vi "Get Delay After FPGA Load.vi"(8 "error in":errorcluster, 11 "scan engine custom device ref in":T1 format="%.0x") -> (0 "error out":errorcluster, 2 "delay after FPGA load (s)":u16, 3 "scan engine custom device ref out":T1 format="%.0x")   [LabVIEW 2019, in "Scan Engine Scripting.lvlib"]
doc: "Returns the <B>delay after FPGA load</B> from a provided Scan Engine custom device reference."
uses:
  Scan Engine Scripting.lvlib
  Shared/Globals/Property Strings.vi
  Shared/SEECD Shared.lvlib
  <vilib>/NI VeriStand/Custom Device API/Custom Device API.lvlib
  <vilib>/NI VeriStand/Custom Device API/Get Item Property (U16).vi
  <vilib>/NI VeriStand/Custom Device API/Custom Device Item Ref.ctl
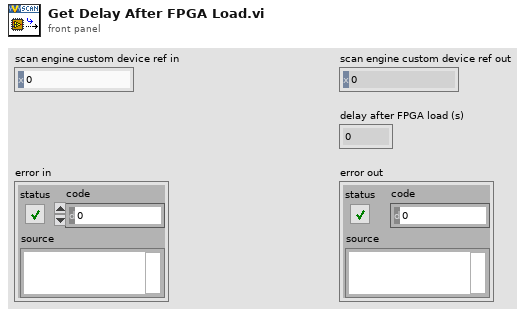
[diagram p1: front panel]
types:
  T1 = typedef "Custom Device API.lvlib/Custom Device Item Ref.ctl" = u64
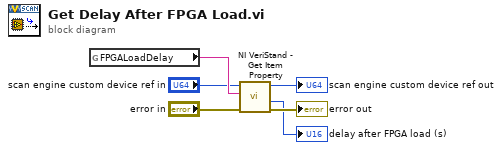
[diagram p0: block diagram]
diagram:
  n1 = global read "Property Strings.vi" "FPGALoadDelay"() -> (w6:string)
  n2 = call-poly <vilib>:"NI VeriStand - Get Item Property.vi"("error in (no error)"="error in", "Property Name"=w6, "Item Ref in"="scan engine custom device ref in") -> ("error out"=→"error out":errorcluster, "Value"=→"delay after FPGA load (s)":u16, "Item Ref out"=→"scan engine custom device ref out":T1)  [unwired: 5 in, 1 out]
